vi "Update Message.vi"(8 "error in (no error)":errorcluster, 10 "Msg":string, 11 "Mesage Display in":refnum<class "Mesage Display.lvclass">) -> (0 "error out":errorcluster, 3 "Mesage Display out":refnum<class "Mesage Display.lvclass">)   [LabVIEW 2020, in "Mesage Display.lvlib" / "Mesage Display.lvclass"]
uses:
  Mesage Display.lvclass
  Mesage Display.lvclass/Mesage Display.ctl
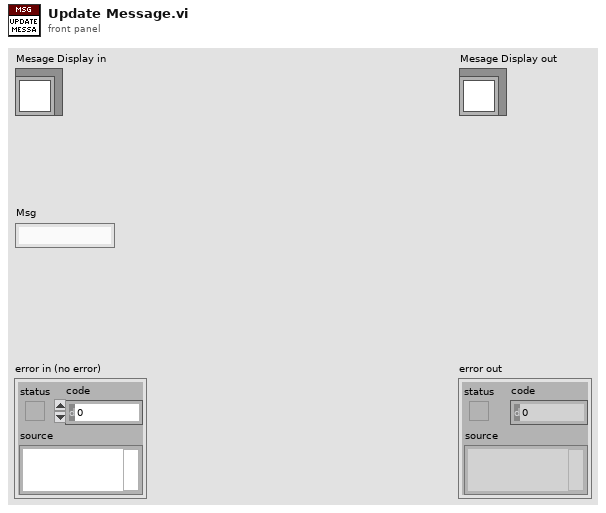
[diagram p1: front panel]
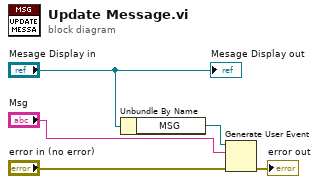
[diagram p0: block diagram]
diagram:
  n1 = Unbundle By Name("Mesage Display in") -> ("MSG"=w2:refnum<user-event>)
  n2 = Generate User Event(user event=w2, event data cluster="Msg", error in="error in (no error)") -> (error out=→"error out":errorcluster)  [unwired: 1 in, 1 out]
  "Mesage Display out" <- "Mesage Display in"
